vi "Stop_LV2.vi"(0 "Stop":bool=TRUE, 11 "error in (no error)":errorcluster, 13 "Operations":T1=enum."Destroy") -> (4 "reference":refnum<user-event>, 15 "error out":errorcluster)   [LabVIEW 2023, in "task_1.lvlib"]
doc: "Stop LV2 variable to use across multiple VIs"
uses:
  task_1.lvlib
  Controls/event_operations.ctl
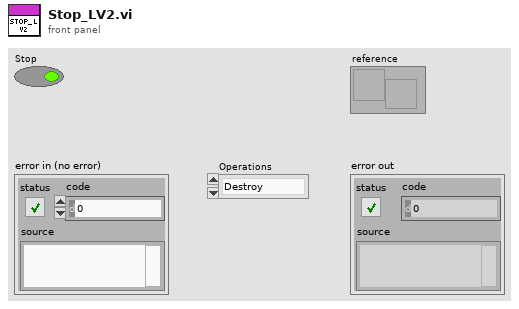
[diagram p1: front panel]
types:
  T1 = typedef "task_1.lvlib/event_operations.ctl" = enum16{"Create", "Generate", "Destroy"}
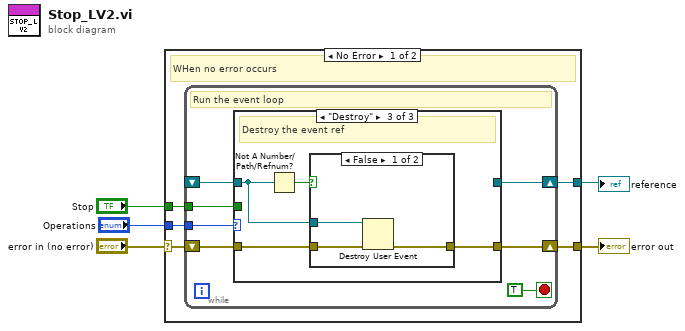
[diagram p0: block diagram]
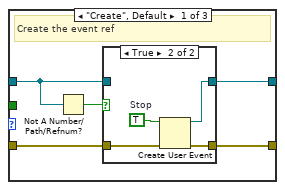
[diagram p2: hidden frame]
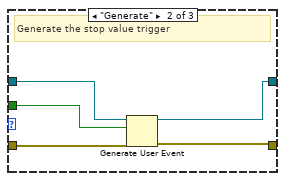
[diagram p4: hidden frame]
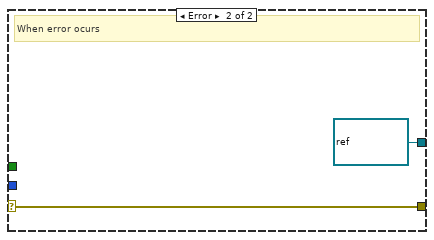
[diagram p6: hidden frame]
diagram:
  n1 = case shown="No Error" "error in (no error)" {
    selector: "error in (no error)" -> [w10 w43]
    tunnel: [w9 w43] -> w4
    tunnel: "Operations" -> [w8 _]
    tunnel: "Stop" -> [w7 _]
    tunnel: [w6 refnum<user-event> refnum ("Stop")] -> w1
    frame No Error {
      # "WHen no error occurs"
      n2 = while {
        shift-right: [w16] -> w9
        shift-left: w10 -> [w17]
        tunnel: w8 -> [w14]
        shift-right: [w13] -> w6
        shift-left: _ -> [w12]
        tunnel: w7 -> [w11]
        stop <- TRUE stop-if-true
        # "Run the event loop"
        n3 = case shown="\"Destroy\"" w14 {
          tunnel: w17 -> [w22 w33 w37]
          tunnel: [w21 w32 w36] -> w16
          tunnel: [w20 w29 _] -> w13
          tunnel: w12 -> [w18 w30 w34]
          tunnel: w11 -> [_ w31 _]
          frame "Create", Default {
            # "Create the event ref"
            n4 = Not A Number/Path/Refnum?(number/path/refnum=w18) -> (NaN/Path/Refnum?=w19:bool)
            n5 = case shown="True" w19 {
              tunnel: w22 -> [w23 w28]
              tunnel: [w23 w27] -> w21
              tunnel: [w24 w25] -> w20
              tunnel: w18 -> [w24 _]
              frame False {
              }
              frame True {
                w26 = TRUE  # Stop
                n6 = Create User Event(user event datatype=w26, error in=w28) -> (user event=w25:refnum<user-event>, error out=w27:errorcluster)
              }
            }
          }
          frame "Generate" {
            # "Generate the stop value trigger"
            n7 = Generate User Event(user event=w30, event data cluster=w31, error in=w33) -> (user event out=w29:refnum<user-event>, error out=w32:errorcluster)  [unwired: 1 in]
          }
          frame "Destroy" {
            # "Destroy the event ref"
            n8 = Not A Number/Path/Refnum?(number/path/refnum=w34) -> (NaN/Path/Refnum?=w35:bool)
            n9 = case shown="False" w35 {
              tunnel: w37 -> [w40 w41]
              tunnel: [w39 w41] -> w36
              tunnel: w34 -> [w38 _]
              frame False {
                n10 = Destroy User Event(user event=w38, error in=w40) -> (error out=w39:errorcluster)
              }
              frame True {
              }
            }
          }
        }
      }
    }
    frame Error {
      # "When error ocurs"
    }
  }
  "error out" <- w4
  "reference" <- w1
